vi "Get VIs in Memory.vi"(3 "error in (no error)":errorcluster) -> (0 "error out":errorcluster, 2 "VIs in Memory":cluster{"vi name":string, "vi path":path}[](array[cluster]))   [LabVIEW 2021, in "Utilities.lvlib"]
doc: "Gathers information about all VIs currently in memory.\n\nFor each VI, it produces this information:\n1) The path to the VI's file.\n2) The size of the data space attached to the VI's front panel. A re-entrant VI has a data space for each usage of the VI. Therefore, this number is not a true reflection of the amount of data a VI is responsible for.\n3&4) The size of the VI's front panel and the number of objects in it; both are zero if the front panel is not currently in memory.\n5&6) Same as above for the block diagram\n7) size of the code generated for this VI.\n8) the VI's description.\n9) The VI's handle.\n10) the indices into the raw data array of this VI's callers\n11) the indices into the raw data array of this VI's callees (subVIs)."
uses:
  Utilities.lvlib
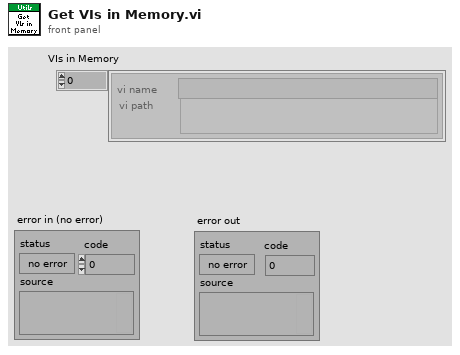
[diagram p1: front panel]
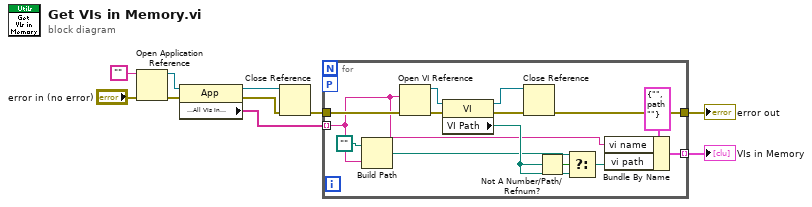
[diagram p0: block diagram]
diagram:
  n1 = Open Application Reference(8:"error in (no error)", 11:"" ("machine name (\"\":  open local reference)")) -> (0:w9:errorcluster, 3:w10:refnum<vi>)  [unwired: 2 in]
  n2 = property class="App"(reference=w10, error in=w9) -> (reference out=w8:refnum<vi>, error out=w7:errorcluster, "Application:All VIs In Memory"=w6:string[])
  n3 = Close Reference(reference=w8, error in (no error)=w7) -> (error out=w4:errorcluster)
  n4 = for {
    tunnel: w6 -> [w15] mode=indexing
    tunnel: [w22] -> w5 mode=indexing
    tunnel: w4 -> [w21]
    tunnel: [w20] -> w2
    workers-P: _ -> [_]
    n5 = Build Path(base path=path "", name or relative path=w15) -> (appended path=w14:path)
    n6 = Open VI Reference(vi path=w15, error in (no error)=w21) -> (vi reference=w24:refnum<vi>, error out=w23:errorcluster)  [unwired: 4 in]
    n7 = property class="VI"(reference=w24, error in=w23) -> (reference out=w12:refnum<vi>, error out=w19:errorcluster, "VI Path"=w17:path)
    n8 = Close Reference(reference=w12, error in (no error)=w19) -> (error out=w20:errorcluster)
    n9 = Not A Number/Path/Refnum?(number/path/refnum=w17) -> (NaN/Path/Refnum?=w18:bool)
    n10 = Select(t=w14, s=w18, f=w17) -> (s? t:f=w16:path)
    n11 = Bundle By Name(cluster=cluster{"vi name":string, "vi path":path} {"vi name"="", "vi path"=path ""}, "vi name"=w15, "vi path"=w16) -> (w22:cluster{"vi name":string, "vi path":path})
  }
  "VIs in Memory" <- w5
  "error out" <- w2
